vi "Pre-Arm.vi"(8 "error in (no error)":errorcluster, 11 "DAQmx Digitizer in":refnum<class "DAQmx Digitizer.lvclass">) -> (0 "error out":errorcluster, 3 "DAQmx Digitizer out":refnum<class "DAQmx Digitizer.lvclass">)   [LabVIEW 2021, in "DAQmx Digitizer.lvclass"]
uses:
  Instruments/Instrument Driver/Instrument Driver.lvclass/Instrument Driver.ctl
  Instruments/Instrument Driver/Write Channel units.vi
  Instruments/Pulse Driver/Pulse Driver.lvclass
  DAQmx Digitizer.lvclass
  DAQmx Digitizer.lvclass/DAQmx Digitizer.ctl
  Instruments/Pulse Driver/Lockin Digitizer Driver/Lockin Digitizer Driver.lvclass
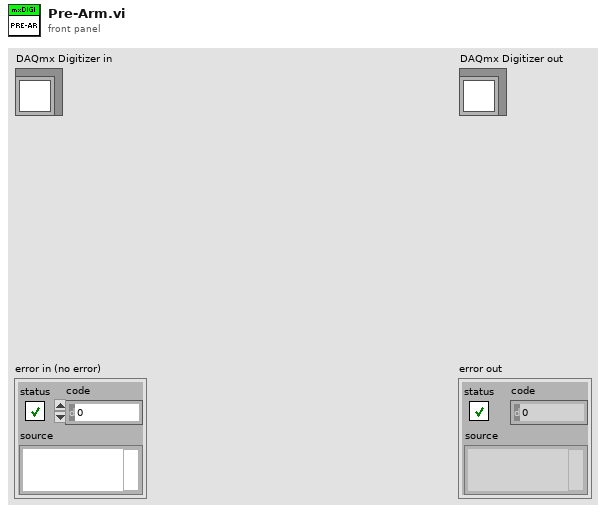
[diagram p1: front panel]
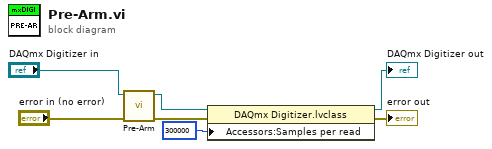
[diagram p0: block diagram]
diagram:
  n1 = call-parent "Pre-Arm.vi"("error in (no error)"="error in (no error)", "Lockin Digitizer Driver in"="DAQmx Digitizer in") -> ("error out"=w3:errorcluster, "Lockin Digitizer Driver out"=w5:refnum<class "DAQmx Digitizer.lvclass">)  [unwired: 8 in]
  n2 = property class="DAQmx Digitizer.lvclass"(reference=w5, error in=w3, "Accessors:Samples per read"=300000) -> (reference out=→"DAQmx Digitizer out":refnum<class "DAQmx Digitizer.lvclass">, error out=→"error out":errorcluster)
